vi "Arrange VIWin - Filter FP Conn Pane Controls.vi"(0 "controls in":refnum<vi>[](array[refnum]), 5 "terminal boundaries":T1[](array[typedef]), 11 "error in":errorcluster) -> (4 "filtered controls":refnum<vi>[](array[refnum]), 6 "filtered terminal boundaries":T1[](array[typedef]), 15 "error out":errorcluster)   [LabVIEW 2017, in "Arrange VI Window.lvlib"]
uses:
  Arrange VI Window.lvlib
  <vilib>/Utility/miscctls.llb/LVRectTypeDef.ctl
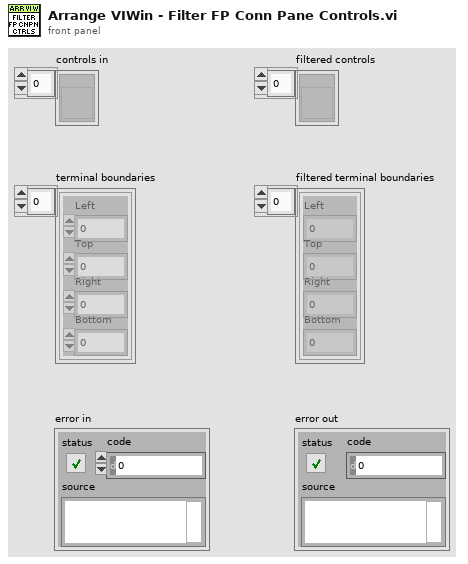
[diagram p1: front panel]
types:
  T1 = typedef "LVRectTypeDef.ctl" = cluster{"Left":i16, "Top":i16, "Right":i16, "Bottom":i16}
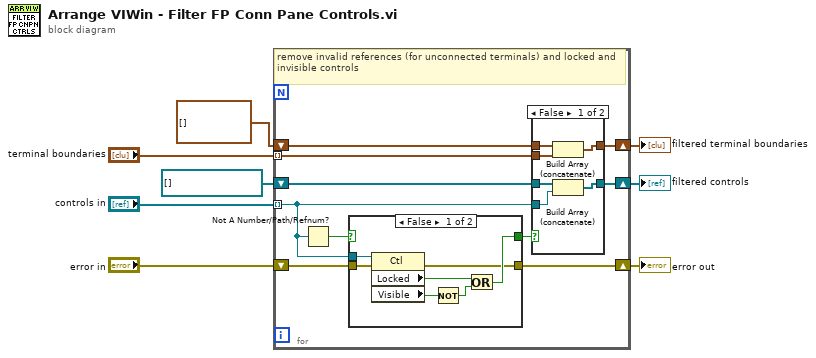
[diagram p0: block diagram]
diagram:
  n1 = for {
    shift-right: [w17] -> w1
    shift-left: refnum<vi>[] [] ("Controls in") -> [w18]
    shift-right: [w15] -> w4
    shift-left: T1[] [] ("TermBnds[]") -> [w16]
    tunnel: "controls in" -> [w10] mode=indexing
    tunnel: "terminal boundaries" -> [w14] mode=indexing
    shift-right: [w12] -> w2
    shift-left: "error in" -> [w11]
    # "remove invalid references (for unconnected terminals) and locked and invisible controls"
    n2 = Not A Number/Path/Refnum?(number/path/refnum=w10) -> (NaN/Path/Refnum?=w9:bool)
    n3 = case shown="False" w9 {
      selector: w9 -> [_ w26]
      tunnel: [w25 w26] -> w13
      tunnel: [w21 w27] -> w12
      tunnel: w11 -> [w20 w27]
      tunnel: w10 -> [w19 _]
      frame False {
        n4 = property class="Ctl"(reference=w19, error in=w20) -> (error out=w21:errorcluster, "Locked"=w22:bool, "Visible"=w23:bool)  [unwired: 1 out]
        n5 = Not(x=w23) -> (.not. x?=w24:bool)
        n6 = Or(x=w22, y=w24) -> (x .or. y?=w25:bool)
      }
      frame True {
      }
    }
    n7 = case shown="False" w13 {
      tunnel: w18 -> [w33 w35]
      tunnel: [w31 w35] -> w17
      tunnel: w16 -> [w32 w34]
      tunnel: [w30 w34] -> w15
      tunnel: w10 -> [w29 _]
      tunnel: w14 -> [w28 _]
      frame False {
        n8 = Build Array (concatenate)(w32, w28) -> (w30:T1[])
        n9 = Build Array (concatenate)(w33, w29) -> (w31:refnum<vi>[])
      }
      frame True {
      }
    }
  }
  "filtered terminal boundaries" <- w4
  "filtered controls" <- w1
  "error out" <- w2
